vi "fit_exponential.vi"(11 "State in":T1={"control refs"={"z offset"=refnum, "laser intensity"=refnum, "XY graph"=refnum}, "error"={"status"=FALSE, "code"=0, "source"=""}, "free-run?"=TRUE, "range (um)"=400, "interpolate?"=FALSE, "settings"={"fix points"=[], "compensation parameters"={"A"=0.0, "lambda"=0.0, "C"=0.0}}} caption="State") -> (3 "State out":T1={"control refs"={"z offset"=refnum, "laser intensity"=refnum, "XY graph"=refnum}, "error"={"status"=FALSE, "code"=0, "source"=""}, "free-run?"=TRUE, "range (um)"=400, "interpolate?"=FALSE, "settings"={"fix points"=[], "compensation parameters"={"A"=0.0, "lambda"=0.0, "C"=0.0}}} caption="State")   [LabVIEW 2010, in "XIntensityCompensation.xctl"]
uses:
  XIntensityCompensation.xctl
  state.ctl
  control_refs.ctl
  settings_cluster.ctl
  data.ctl
  <vilib>/Analysis/6fits.llb/Curve Fitting Criteria.ctl
  <vilib>/Analysis/NI_AALPro.lvlib
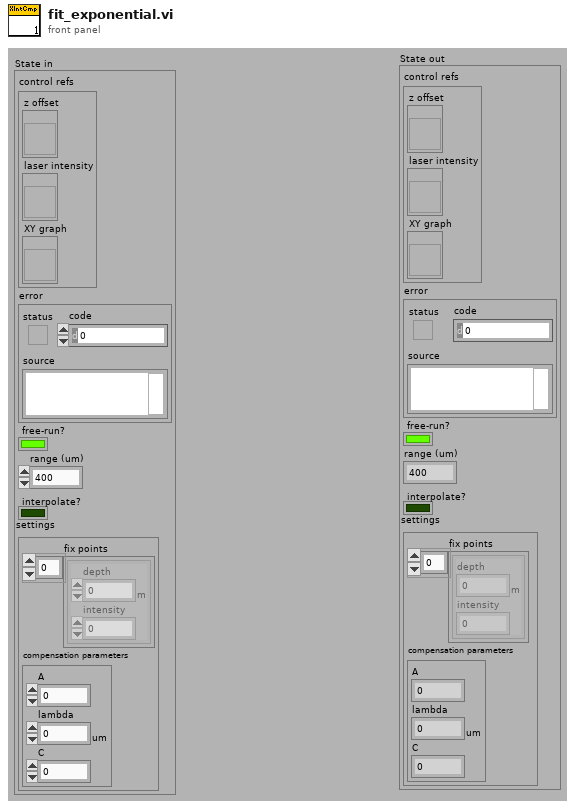
[diagram p1: front panel]
types:
  T1 = typedef "XIntensityCompensation.xctl/state.ctl" = cluster{"control refs":T2, "error":errorcluster, "free-run?":bool, "range (um)":i32, "interpolate?":bool, "settings":T3}
  T2 = typedef "XIntensityCompensation.xctl/control_refs.ctl" = cluster{"z offset":refnum<vi>, "laser intensity":refnum<vi>, "XY graph":refnum<vi>}
  T3 = typedef "XIntensityCompensation.xctl/settings_cluster.ctl" = cluster{"fix points":cluster{"depth":dbl[unit], "intensity":dbl}[], "compensation parameters":T4}
  T4 = typedef "XIntensityCompensation.xctl/data.ctl" = cluster{"A":dbl, "lambda":dbl[unit], "C":dbl}
  T5 = typedef "NI_AALPro.lvlib/Curve Fitting Criteria.ctl" = u16
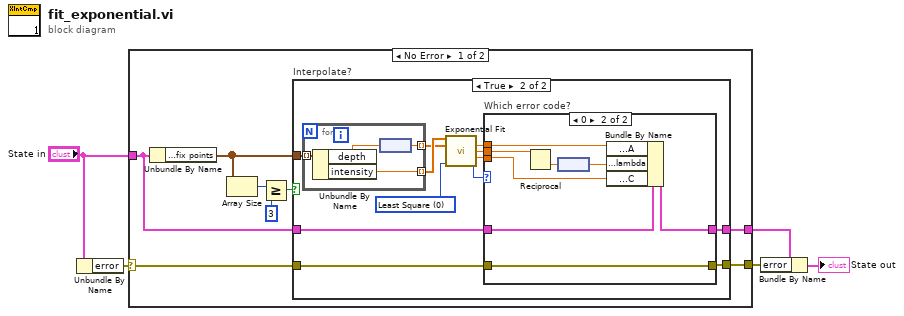
[diagram p0: block diagram]
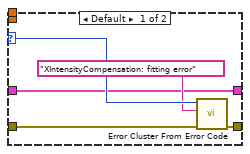
[diagram p3: hidden frame]
diagram:
  n1 = Unbundle By Name("State in") -> ("error"=w1:errorcluster)
  n2 = case shown="No Error" w1 {
    selector: w1 -> [w7 w46]
    tunnel: [w10 w45] -> w5
    tunnel: [w9 w46] -> w3
    tunnel: "State in" -> [w6 w45]
    frame No Error {
      n3 = Unbundle By Name(w6) -> ("settings.fix points"=w13:cluster{"depth":dbl[unit], "intensity":dbl}[])
      n4 = Array Size(array=w13) -> (size(s)=w12:i32)
      n5 = Greater Or Equal?(x=w12, y=3) -> (x >= y?=w8:bool)
      n6 = case "Interpolate?" shown="True" w8 {
        tunnel: w13 -> [_ w27]
        tunnel: w7 -> [w15 w26]
        tunnel: [w15 w25] -> w9
        tunnel: w6 -> [w14 w17]
        tunnel: [w14 w16] -> w10
        frame False {
        }
        frame True {
          w22 = T5 0 items=["Least Square", "Least Absolute Residual", "Bisquare"] ("method")
          n7 = for {
            tunnel: w27 -> [w44] mode=indexing
            tunnel: [w43] -> w24 mode=indexing
            tunnel: [w42] -> w23 mode=indexing
            n8 = Unbundle By Name(w44) -> ("depth"=w41:dbl[unit], "intensity"=w43:dbl)
            n9 = node(w41) -> (w42:dbl)
          }
          n10 = call <vilib>:"Exponential Fit.vi"("Y"=w24, "X"=w23, "method"=w22) -> ("amplitude"=w20:dbl, "damping"=w19:dbl, "offset"=w21:dbl, "error"=w18:i32)  [unwired: 7 in, 2 out]
          n11 = case "Which error code?" shown="0" w18 {
            selector: w18 -> [w32 _]
            tunnel: w21 -> [_ w38]
            tunnel: w20 -> [_ w39]
            tunnel: w19 -> [_ w37]
            tunnel: w26 -> [w31 w40]
            tunnel: [w29 w40] -> w25
            tunnel: w17 -> [w28 w36]
            tunnel: [w28 w33] -> w16
            frame Default {
              n12 = call <vilib>:"Error Cluster From Error Code.vi"("error in (no error)"=w31, "error message (\"\")"="XIntensityCompensation: fitting error" ("error message (\"\")"), "error code (0)"=w32) -> ("error out"=w29:errorcluster)  [unwired: 6 in]
            }
            frame 0 {
              n13 = Reciprocal(x=w37) -> (1/x=w34:dbl)
              n14 = node(w34) -> (w35:dbl[unit])
              n15 = Bundle By Name(cluster=w36, "settings.compensation parameters.A"=w39, "settings.compensation parameters.lambda"=w35, "settings.compensation parameters.C"=w38) -> (w33:T1)
            }
          }
        }
      }
    }
    frame Error {
    }
  }
  n16 = Bundle By Name(cluster=w5, "error"=w3) -> (→"State out":T1)
